vi "Get or Add Columns.vi"(8 "error in":errorcluster, 10 "Sheet Name":string, 11 "SpreadsheetDoc in":refnum<k24>) -> (0 "error out":errorcluster, 2 "Columns":refnum<k24>, 3 "SpreadsheetDoc out":refnum<k24>)   [LabVIEW 2019, in "Open Xml.lvlib"]
uses:
  Open Xml.lvlib
  D:/git/Open-Xml-LabVIEW/Source/DocumentFormat.OpenXml.dll
  DocumentFormat.OpenXml.dll
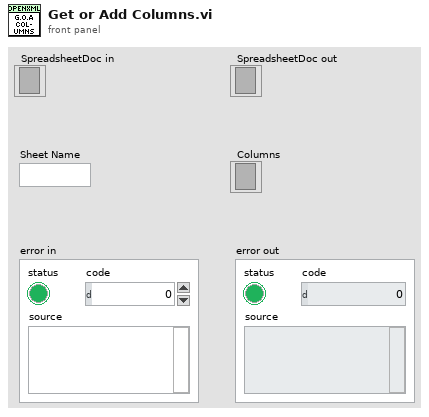
[diagram p1: front panel]
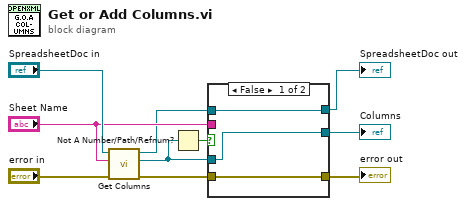
[diagram p0: block diagram]
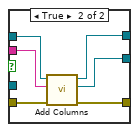
[diagram p2: hidden frame]
diagram:
  n1 = call "Get Columns.vi"("error in"="error in", "Sheet Name"="Sheet Name", "SpreadsheetDoc in"="SpreadsheetDoc in") -> ("error out"=w7:errorcluster, "Columns"=w1:refnum<k24>, "SpreadsheetDoc out"=w4:refnum<k24>)  [unwired: 6 in]
  n2 = Not A Number/Path/Refnum?(number/path/refnum=w1) -> (NaN/Path/Refnum?=w8:bool)
  n3 = case shown="False" w8 {
    tunnel: w7 -> [w13 w19]
    tunnel: [w13 w15] -> w6
    tunnel: "Sheet Name" -> [_ w18]
    tunnel: w4 -> [w12 w17]
    tunnel: [w12 w16] -> w3
    tunnel: [w11 w14] -> w2
    tunnel: w1 -> [w11 _]
    frame False {
    }
    frame True {
      n4 = call "Add Columns.vi"("error in"=w19, "Sheet Name"=w18, "SpreadsheetDoc in"=w17) -> ("error out"=w15:errorcluster, "Columns"=w14:refnum<k24>, "SpreadsheetDoc out"=w16:refnum<k24>)  [unwired: 6 in]
    }
  }
  "error out" <- w6
  "SpreadsheetDoc out" <- w3
  "Columns" <- w2
